vi "chart set rotation.vi"(8 "error in (no error)":errorcluster, 10 "rotation":u16, 11 "chart":u32) -> (0 "error out":errorcluster)   [LabVIEW 2015, in "xlsxwriter.lvlib"]
doc: "void chart_set_rotation(lxw_chart chart, uint16_t rotation);"
uses:
  xlsxwriter.lvlib
  xlsxwriter.dll
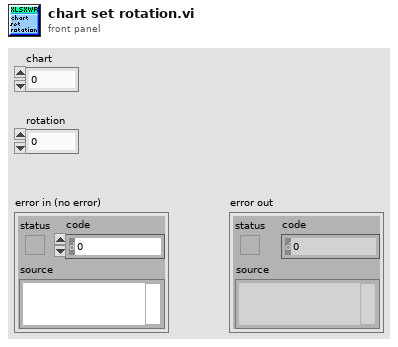
[diagram p1: front panel]
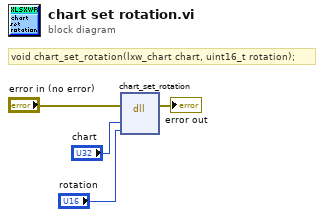
[diagram p0: block diagram]
diagram:
  # "void chart_set_rotation(lxw_chart chart, uint16_t rotation);"
  n1 = dll-call lib="C:/Users/WDAGUtilityAccount/Desktop/lv_vis_added_cell/xlsxwriter.*" fn="chart_set_rotation"(error in="error in (no error)", "chart"="chart", "rotation"="rotation") -> (error out=→"error out":errorcluster)  [unwired: 5 in, 1 out]
